vi "2d_array.vi"() -> ()   [LabVIEW 2017]
uses:
  support/my_global.vi
panel:
  out "size(s)":i32[](array[numeric])
  out "Array":dbl[][](array[numeric])
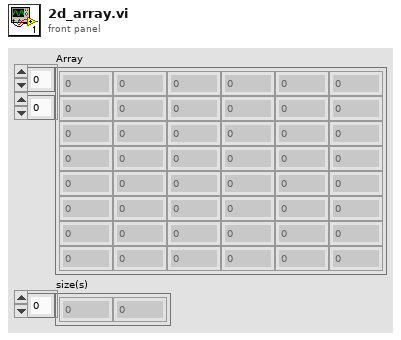
[diagram p1: front panel]
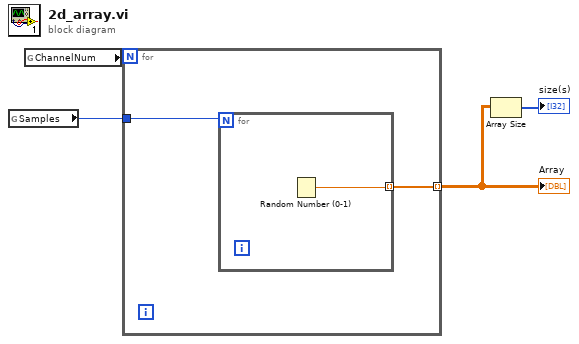
[diagram p0: block diagram]
diagram:
  n1 = global read "my_global.vi" "Samples"() -> (w1:u32)
  n2 = global read "my_global.vi" "ChannelNum"() -> (w2:u32)
  n3 = for {
    N: w2 -> [_]
    tunnel: [w6] -> w4 mode=indexing
    tunnel: w1 -> [w5]
    n4 = for {
      N: w5 -> [_]
      tunnel: [w7] -> w6 mode=indexing
      n5 = Random Number (0-1)() -> (number: 0 to 1=w7:dbl)
    }
  }
  "Array" <- w4
  n6 = Array Size(array=w4) -> (size(s)=→"size(s)":i32[])
